vi "activeGalvo.vi"() -> (0 "error out":errorcluster, 1 "Galvo-resource out":T1)   [LabVIEW 2011]
uses:
  Drivers/SIAM/SIAM-send.ctl
panel:
  # "analog=? valid taski ID >String\ndigital= valid VISA?!>FlattenedString\ndigital-siam, data=not used"
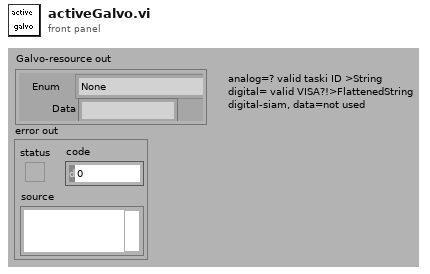
[diagram p1: front panel]
types:
  T1 = cluster{"Enum":enum16{"None", "DSP-on serial port", "Analog out", "SIAM-withDSiam"}, "Data":string}
  T2 = enum16{"None/#Datasets", "Clear", "TagValueOf#", "AddValues", "ReadValue", "ChangeValue", "Get all"}
  T3 = enum16{"None", "DSP-on serial port", "Analog out"}
  T4 = enum16{"None", "DSP-on serial port", "Analog out", "SIAM-withDSiam"}
  T5 = typedef "SIAM-send.ctl" = enum16{"validID", "storeID", "enable", "rundirect", "sendlist", "run", "stop", "readRegister", "sendValue", "storeStatus"}
  T6 = cluster{"Enum":enum16{"None", "DSP-on serial port", "Analog out", "SIAM-withDSiam"}, "data string":string}
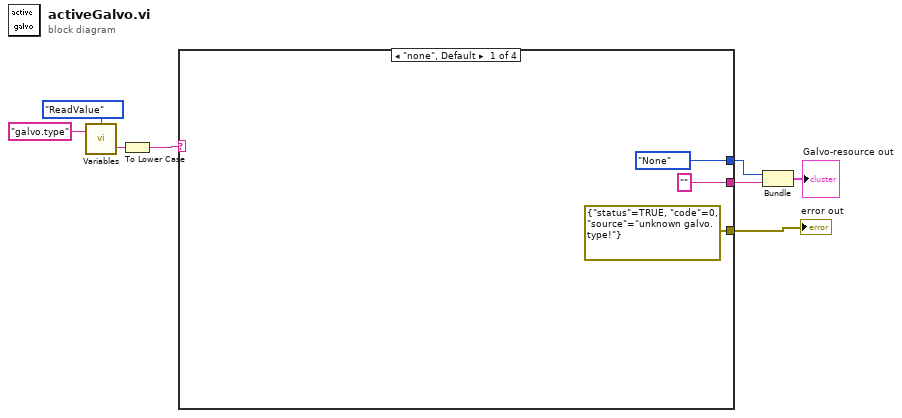
[diagram p0: block diagram]
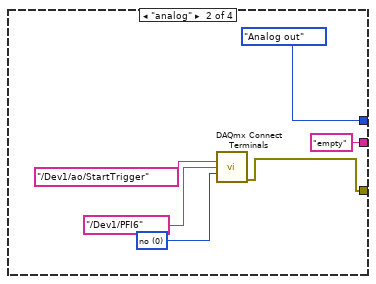
[diagram p2: hidden frame]
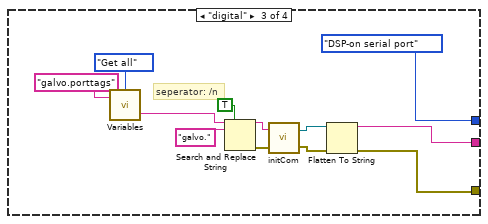
[diagram p3: hidden frame]
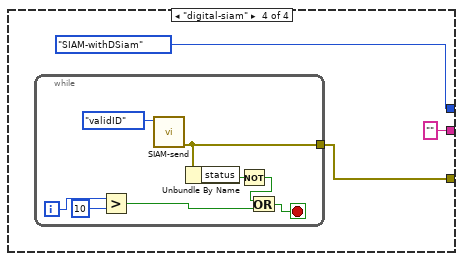
[diagram p4: hidden frame]
diagram:
  n1 = call "Variables.vi"("Tag in"="galvo.type", "Command"=T2."ReadValue") -> ("value out"=w3:string)  [unwired: 1 in, 2 out]
  n2 = To Lower Case(string=w3) -> (all lower case string=w1:string)
  n3 = case shown="\"none\", Default" w1 {
    tunnel: [T3."None" ("Enum") T3."Analog out" ("Enum") T3."DSP-on serial port" ("Enum") T4."SIAM-withDSiam" ("Enum")] -> w8
    tunnel: ["" ("ValueText") "empty" w28 "" ("data string")] -> w7
    tunnel: [errorcluster {"status"=TRUE, "code"=0, "source"="unknown galvo.type!"} ("error out") w14 w18 w30] -> w2
    frame "none", Default {
    }
    frame "analog" {
      w15 = 0 items=["no", "yes"] ("invert polarity")
      n4 = call <vilib>:"DAQmx Connect Terminals.vi"("source terminal"=tag "/Dev1/ao/StartTrigger", "destination terminal"=tag "/Dev1/PFI6", "invert polarity"=w15) -> ("error out"=w14:errorcluster)  [unwired: 1 in, 11 out]
    }
    frame "digital" {
      # "seperator: /n"
      n5 = call "Variables.vi"("Tag in"="galvo.porttags", "Command"=T2."Get all") -> ("value out"=w25:string)  [unwired: 1 in, 2 out]
      n6 = Search and Replace String(replace all?=TRUE ("replace all? (F)"), input string=w25, search string="galvo.") -> (result string=w22:string, error out=w20:errorcluster)  [unwired: 1 in, 6 out]
      n7 = call "initCom.vi"("error in (no error)"=w20, "String port=\"\" baud=\"\" etc"=w22) -> ("error out"=w19:errorcluster, "VISA resource name"=w21:refnum<visa-resource-name>)
      n8 = Flatten To String(anything=w21, error in (no error)=w19) -> (data string=w28:string, error out=w18:errorcluster)  [unwired: 3 out]
    }
    frame "digital-siam" {
      n9 = while {
        tunnel: [w39] -> w30
        i -> [w38]
        stop <- w33 stop-if-true
        n10 = Greater?(x=w38, y=10) -> (0:w34:bool)
        n11 = call "SIAM-send.vi"("command"=SIAM-send."validID") -> ("error out"=w39:errorcluster)  [unwired: 9 in, 1 out]
        n12 = Unbundle By Name(w39) -> ("status"=w36:bool)
        n13 = Not(x=w36) -> (.not. x?=w35:bool)
        n14 = Or(x=w35, y=w34) -> (x .or. y?=w33:bool)
      }
    }
  }
  "error out" <- w2
  n15 = Bundle("Enum"=w8, "data string"=w7) -> (→"Galvo-resource out":T6)  [unwired: 1 out]
